vi "EOL CAN_Download CAL.vi"(4 "Download CAL Progress":refnum<vi>, 5 "Download CAL Time":refnum<vi>, 6 "ODX File Path":path, 7 "Tester":refnum<k21>, 8 "Error String":string, 9 "Glass?":bool=TRUE, 10 "Read Session in":refnum<k21>, 11 "DSC Write Session in":refnum<k21>) -> (1 "Error String Out":string, 2 "TxRx Data":string[][](array[string]), 3 "Response Good?":bool)   [LabVIEW 2014]
panel:
  in  "stop 2":bool
  in  "stop":bool
  out "error out":errorcluster
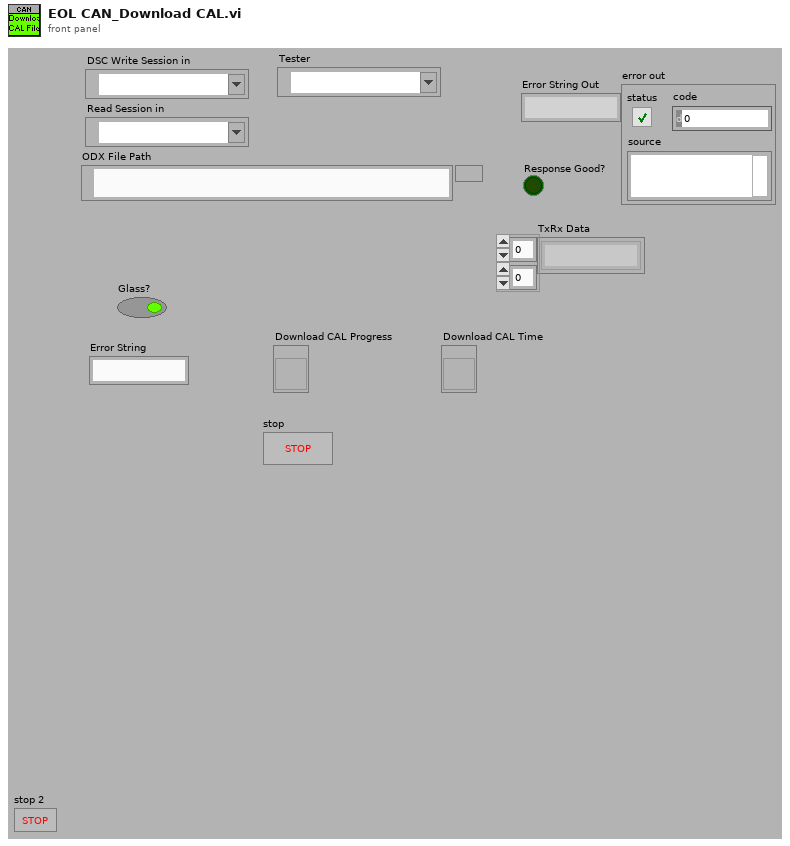
[diagram p1: front panel]
types:
  T1 = cluster{"DSC Write Session in":refnum<k21>, "Read Session in":refnum<k21>, "Error String":string, "Response Good?":bool, "Glass?":bool, "TxRx Data":string[][], "ODX File Path":path, "Flash Data Array":u8[], "Download CAL Progress":refnum<vi>, "Download CAL Time":refnum<vi>, "millisecond timer value":u32}
  T2 = typedef "Diagnose_SA2_Rechnenbefehl.ctl" = cluster{"Operation":T3, "Wert":u32}
  T3 = typedef "Diagnose_SA2_Operation_ENUM.ctl" = enum16{"RSL", "RSR", "ADD", "SUB", "EOR", "Durchläufe", "NEXT", "BCC", "BRA", "Fertig"}
  T4 = typedef "XNET Frame CAN.ctl" = cluster{"timestamp":timestamp, "payload":u8[], "identifier":u32, "type":T5, "extended?":bool, "echo?":bool}
  T5 = typedef "XNET Frame Type CAN.ctl" = u8
  T6 = cluster{"Start Adress":u8[], "Block Size":u8[], "Checksum":u8[]}
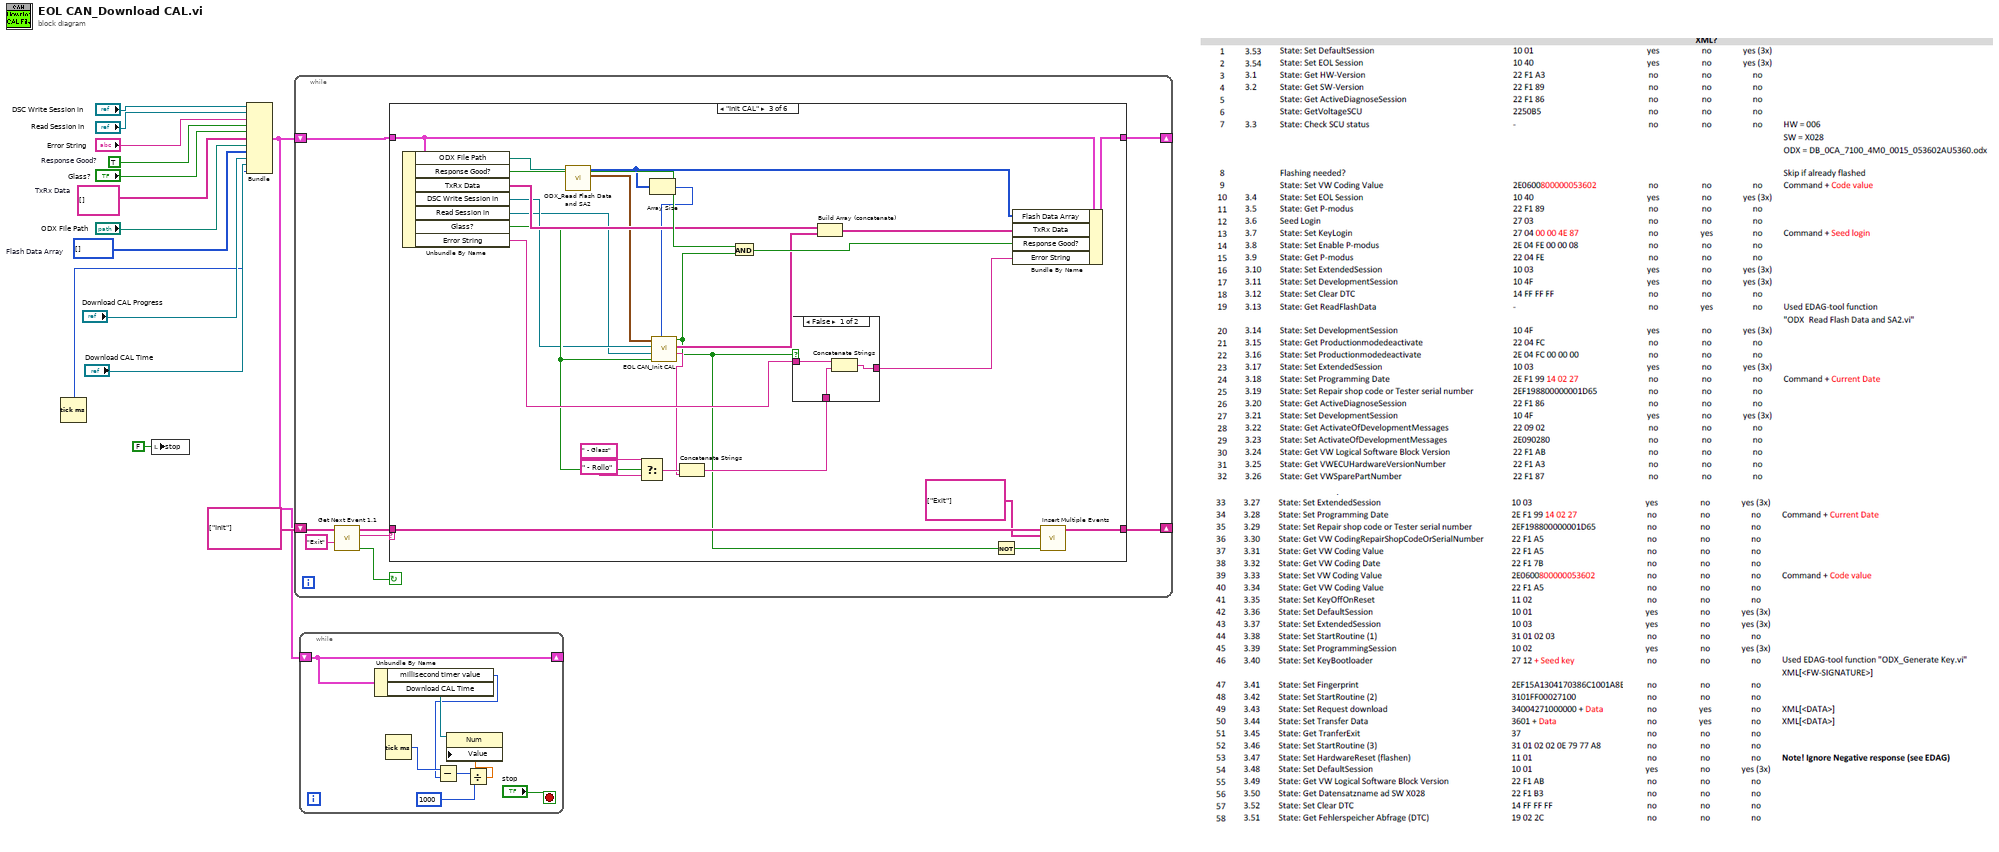
[diagram p0: block diagram]
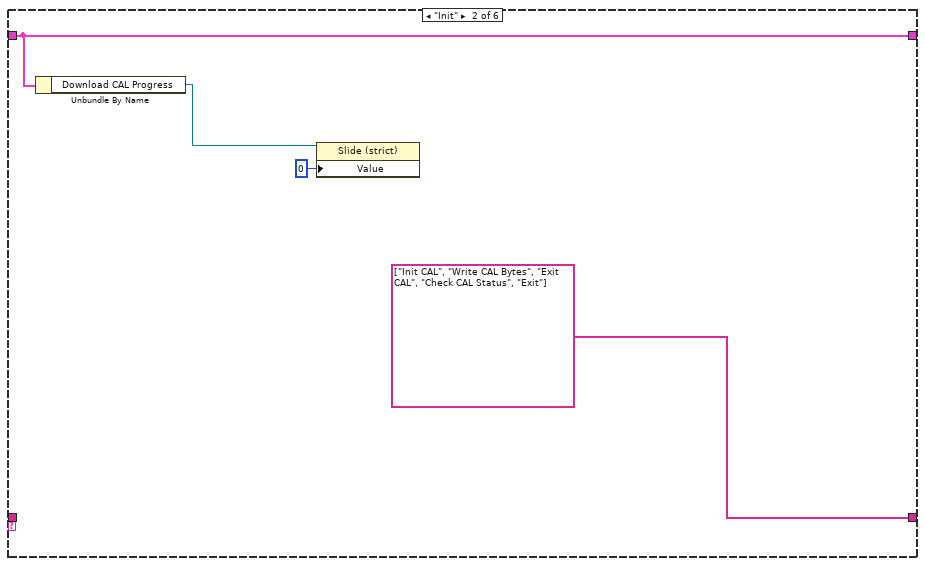
[diagram p3: hidden frame]
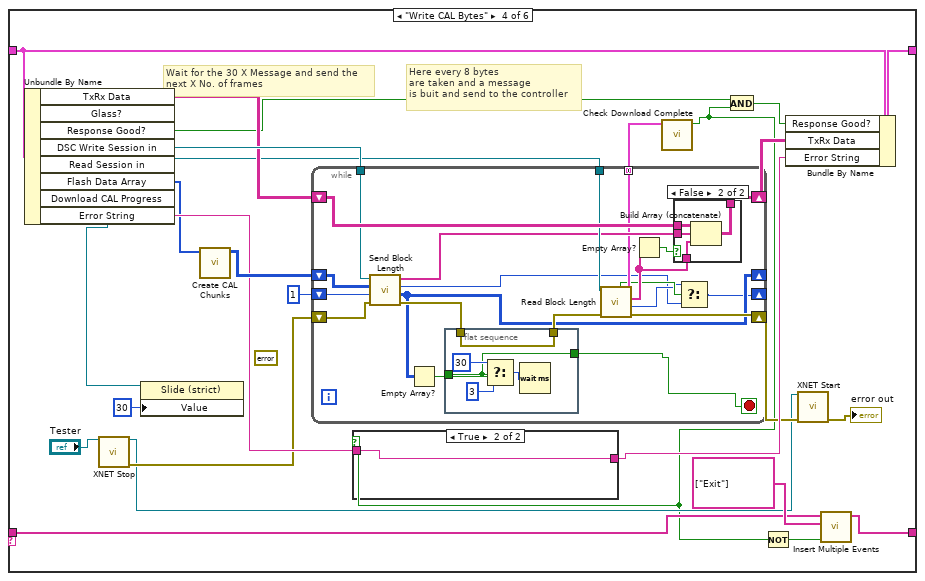
[diagram p5: hidden frame]
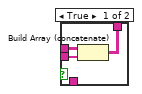
[diagram p6: hidden frame]
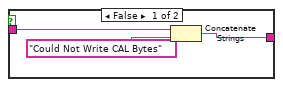
[diagram p7: hidden frame]
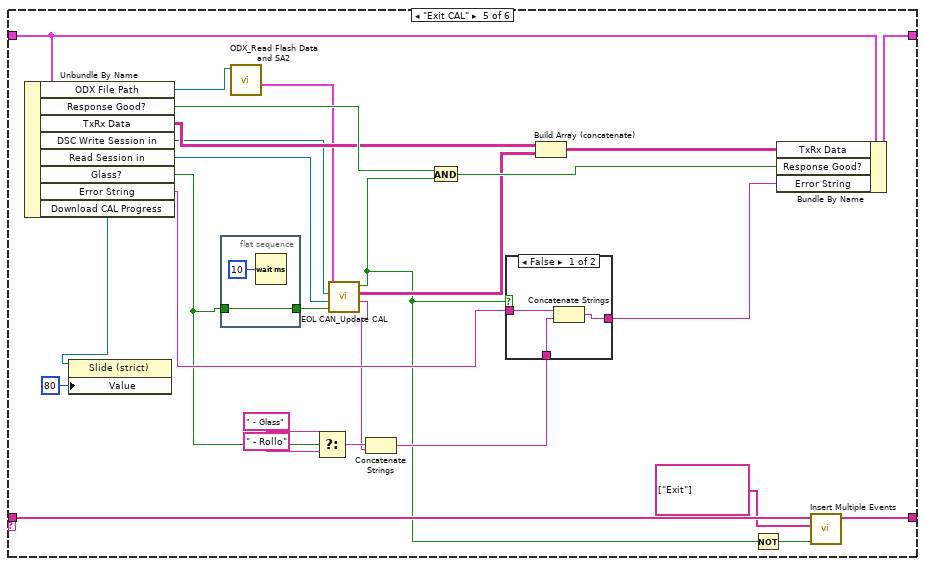
[diagram p8: hidden frame]
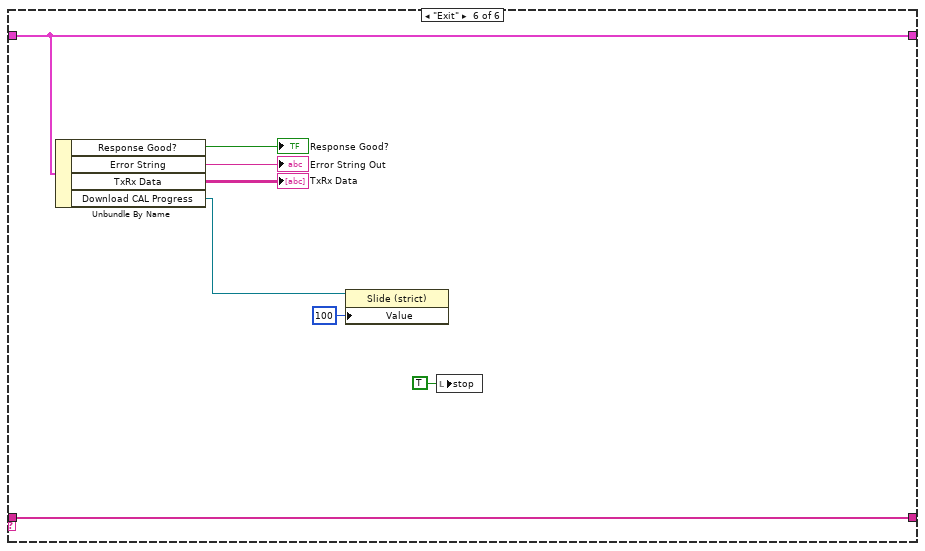
[diagram p10: hidden frame]
diagram:
  w6 = u8[] []  # Flash Data Array
  w10 = string[][] []  # TxRx Data
  w12 = TRUE  # Response Good?
  n1 = Tick Count (ms)() -> (millisecond timer value=w3:u32)
  n2 = local write "stop"(FALSE ("stop")) -> ()
  n3 = Bundle("DSC Write Session in"="DSC Write Session in", "Read Session in"="Read Session in", "Error String"="Error String", "Response Good?"=w12, "Glass?"="Glass?", "TxRx Data"=w10, "ODX File Path"="ODX File Path", "Flash Data Array"=w6, "Download CAL Progress"="Download CAL Progress", "Download CAL Time"="Download CAL Time", "millisecond timer value"=w3) -> (w2:T1)  [unwired: 1 in]
  n4 = while {
    shift-right: [w20] -> _
    shift-left: string[] ["Init"] ("event queue out") -> [w19]
    shift-right: [w18] -> _
    shift-left: w2 -> [w15]
    stop <- w22 continue-if-true
    n5 = call "Get Next Event 1.1.vi"("Exit Event"="Exit", "event queue in"=w19) -> ("Condition (Exit:F)"=w22:bool, "next event"=w16:string, "event queue out"=w21:string[])  [unwired: 6 in, 1 out]
    n6 = case shown="\"Init CAL\"" w16 {
      tunnel: w21 -> [w24 _ w43 w72 w145 w162]
      tunnel: [w24 string[] ["Init CAL", "Write CAL Bytes", "Exit CAL", "Check CAL Status", "Exit"] ("event queue out") w44 w73 w146 w162] -> w20
      tunnel: w15 -> [w23 w25 w53 w84 w148 w161]
      tunnel: [w23 w25 w51 w83 w147 w161] -> w18
      frame "Error", Default {
      }
      frame "Init" {
        n7 = Unbundle By Name(w25) -> ("Download CAL Progress"=w27:refnum<vi>)
        n8 = property class="Slide (strict)"(reference=w27, "Value"=u8 0) -> ()  [unwired: 1 in, 2 out]
      }
      frame "Init CAL" {
        n9 = Unbundle By Name(w53) -> ("ODX File Path"=w38:path, "Response Good?"=w54:bool, "TxRx Data"=w41:string[][], "DSC Write Session in"=w32:refnum<k21>, "Read Session in"=w31:refnum<k21>, "Glass?"=w33:bool, "Error String"=w50:string)
        n10 = call "ODX_Read Flash Data and SA2.vi"("ODX File Path"=w38) -> ("SA2 Operator"=w39:T2[], "Flash Data Array"=w30:u8[])  [unwired: 7 in, 2 out]
        n11 = Select(t=" - Glass" ("Error Description"), s=w33, f=" - Rollo" ("Error Description")) -> (s? t:f=w48:string)
        n12 = Array Size(array=w30) -> (size(s)=w29:i32)
        n13 = call "EOL CAN_Init CAL.vi"("Flash Size"=w29, "Glass?"=w33, "Read Session in"=w31, "DSC Write Session in"=w32, "SA2 Operator"=w39) -> ("Error String Out"=w36:string, "TxRx Data"=w37:string[][], "Response Good?"=w35:bool)  [unwired: 4 in]
        n14 = Concatenate Strings(w48, w36) -> (w45:string)
        n15 = And(x=w54, y=w35) -> (x .and. y?=w52:bool)
        n16 = case shown="False" w35 {
          tunnel: w50 -> [w56 w58]
          tunnel: [w57 w58] -> w49
          tunnel: w45 -> [w55 _]
          frame False {
            n17 = Concatenate Strings(w56, w55) -> (w57:string)
          }
          frame True {
          }
        }
        n18 = Build Array (concatenate)(w41, w37) -> (w40:string[][])
        n19 = Not(x=w35) -> (.not. x?=w34:bool)
        n20 = Bundle By Name(cluster=w53, "Flash Data Array"=w30, "TxRx Data"=w40, "Response Good?"=w52, "Error String"=w49) -> (w51:T1)
        n21 = call "Insert Multiple Events.vi"("Insert all? (T)"=w34, "Events to Insert"=string[] ["Exit"], "Event queue in"=w43) -> ("Event queue out"=w44:string[])  [unwired: 4 in]
      }
      frame "Write CAL Bytes" {
        (unwired) errorcluster {"status"=FALSE, "code"=0, "source"=""} ("error out 2")
        # "Wait for the 30 X Message and send the\nnext X No. of frames"
        # "Here every 8 bytes\nare taken and a message\nis buit and send to the controller"
        n22 = Unbundle By Name(w84) -> ("TxRx Data"=w81:string[][], "Response Good?"=w77:bool, "DSC Write Session in"=w82:refnum<k21>, "Read Session in"=w76:refnum<k21>, "Flash Data Array"=w59:u8[], "Download CAL Progress"=w70:refnum<vi>, "Error String"=w69:string)  [unwired: 1 out]
        n23 = call <vilib>:"XNET Stop.vi"("session in"="Tester") -> ("session out"=w64:refnum<k21>, "error out"=w66:errorcluster)  [unwired: 13 in]
        n24 = property class="Slide (strict)"(reference=w70, "Value"=u8 30) -> ()  [unwired: 1 in, 2 out]
        n25 = call "Create CAL Chunks.vi"("Flash Data Array"=w59) -> ("Array 2"=w80:u8[][])  [unwired: 10 in]
        n26 = while {
          tunnel: w82 -> [w103]
          shift-right: [w104] -> w79
          shift-left: w81 -> [w105]
          tunnel: w76 -> [w102]
          tunnel: [w100] -> w62 mode=concatenating
          shift-right: [w95] -> w65
          shift-left: w66 -> [w94]
          shift-right: [w86] -> _
          shift-left: u16 1 ("Block Size") -> [w93]
          shift-right: [w89] -> _
          shift-left: w80 -> [w91]
          stop <- w90 stop-if-true
          n27 = call "Send Block Length.vi"("error in (no error)"=w94, "Block Size In"=w93, "Array in"=w91, "Refnum in"=w103) -> ("error out"=w97:errorcluster, "Array Out"=w89:u8[][], "Block Size Out"=w85:u32, "Array out"=w101:string[])  [unwired: 4 in]
          n28 = Empty Array?(array=w89) -> (empty?=w92:bool)
          n29 = flat-sequence {
            tunnel: w97 -> [w110]
            tunnel: [w110] -> w96
            tunnel: w92 -> [w106]
            tunnel: [w106] -> w90
            frame #0 {
              n30 = Select(t=u32 30, s=w106, f=u32 3 ("milliseconds to wait")) -> (s? t:f=w109:u32)
              n31 = Wait (ms)(milliseconds to wait=w109) -> ()  [unwired: 1 out]
            }
          }
          n32 = call "Read Block Length.vi"("error in (no error)"=w96, "Refnum in"=w102) -> ("error out"=w95:errorcluster, "Block Size"=w87:u16, "Array"=w98:string[], "data"=w100:T4[], "Flow Control?"=w88:bool)  [unwired: 5 in]
          n33 = Empty Array?(array=w98) -> (empty?=w99:bool)
          n34 = case shown="False" w99 {
            tunnel: w105 -> [w113 w117]
            tunnel: [w112 w116] -> w104
            tunnel: w101 -> [w111 w115]
            tunnel: w98 -> [_ w114]
            frame True {
              n35 = Build Array (concatenate)(w113, w111) -> (w112:string[][])
            }
            frame False {
              n36 = Build Array (concatenate)(w117, w115, w114) -> (w116:string[][])
            }
          }
          n37 = Select(t=w87, s=w88, f=w85) -> (s? t:f=w86:u32)
        }
        n38 = call "Check Download Complete.vi"("data"=w62) -> ("Boolean"=w61:bool)  [unwired: 10 in]
        n39 = case shown="True" w61 {
          tunnel: w69 -> [w120 w121]
          tunnel: [w118 w121] -> w68
          frame False {
            n40 = Concatenate Strings(w120, "Could Not Write CAL Bytes" ("string")) -> (w118:string)
          }
          frame True {
          }
        }
        n41 = And(x=w77, y=w61) -> (x .and. y?=w78:bool)
        n42 = Not(x=w61) -> (.not. x?=w74:bool)
        n43 = Bundle By Name(cluster=w84, "Response Good?"=w78, "TxRx Data"=w79, "Error String"=w68) -> (w83:T1)
        n44 = call <vilib>:"XNET Start.vi"("session in"=w64, "error in (no error)"=w65) -> ("error out"=→"error out":errorcluster)  [unwired: 12 in, 1 out]
        n45 = call "Insert Multiple Events.vi"("Insert all? (T)"=w74, "Events to Insert"=string[] ["Exit"], "Event queue in"=w72) -> ("Event queue out"=w73:string[])  [unwired: 4 in]
      }
      frame "Exit CAL" {
        n46 = Unbundle By Name(w148) -> ("ODX File Path"=w127:path, "Response Good?"=w144:bool, "TxRx Data"=w135:string[][], "DSC Write Session in"=w132:refnum<k21>, "Read Session in"=w131:refnum<k21>, "Glass?"=w125:bool, "Error String"=w142:string, "Download CAL Progress"=w122:refnum<vi>)
        n47 = property class="Slide (strict)"(reference=w122, "Value"=u8 80) -> ()  [unwired: 1 in, 2 out]
        n48 = flat-sequence {
          tunnel: w125 -> [w149]
          tunnel: [w149] -> w124
          frame #0 {
            n49 = Wait (ms)(milliseconds to wait=u32 10) -> ()  [unwired: 1 out]
          }
        }
        n50 = call "ODX_Read Flash Data and SA2.vi"("ODX File Path"=w127) -> ("Download Parameter"=w126:T6)  [unwired: 7 in, 3 out]
        n51 = Select(t=" - Glass" ("Error Description"), s=w125, f=" - Rollo" ("Error Description")) -> (s? t:f=w140:string)
        n52 = call "EOL CAN_Update CAL.vi"("Glass?"=w124, "Read Session in"=w131, "DSC Write Session in"=w132, "Download Parameter"=w126) -> ("Error String Out"=w129:string, "TxRx Data"=w130:string[][], "Response Good?"=w128:bool)  [unwired: 5 in]
        n53 = Concatenate Strings(w140, w129) -> (w137:string)
        n54 = And(x=w144, y=w128) -> (x .and. y?=w143:bool)
        n55 = case shown="False" w128 {
          tunnel: w142 -> [w152 w154]
          tunnel: [w153 w154] -> w141
          tunnel: w137 -> [w151 _]
          frame False {
            n56 = Concatenate Strings(w152, w151) -> (w153:string)
          }
          frame True {
          }
        }
        n57 = Build Array (concatenate)(w135, w130) -> (w134:string[][])
        n58 = Not(x=w128) -> (.not. x?=w133:bool)
        n59 = Bundle By Name(cluster=w148, "TxRx Data"=w134, "Response Good?"=w143, "Error String"=w141) -> (w147:T1)
        n60 = call "Insert Multiple Events.vi"("Insert all? (T)"=w133, "Events to Insert"=string[] ["Exit"], "Event queue in"=w145) -> ("Event queue out"=w146:string[])  [unwired: 4 in]
      }
      frame "Exit" {
        n61 = Unbundle By Name(w161) -> ("Response Good?"=→"Response Good?":bool, "Error String"=→"Error String Out":string, "TxRx Data"=→"TxRx Data":string[][], "Download CAL Progress"=w156:refnum<vi>)
        n62 = property class="Slide (strict)"(reference=w156, "Value"=u8 100) -> ()  [unwired: 1 in, 2 out]
        n63 = local write "stop"(TRUE ("stop")) -> ()
      }
    }
  }
  n64 = while {
    shift-right: [w165] -> _
    shift-left: w2 -> [w165]
    stop <- "stop" stop-if-true
    n65 = Unbundle By Name(w165) -> ("millisecond timer value"=w164:u32, "Download CAL Time"=w169:refnum<vi>)
    n66 = Tick Count (ms)() -> (millisecond timer value=w166:u32)
    n67 = Subtract(x=w166, y=w164) -> (x-y=w167:u32)
    n68 = Divide(x=w167, y=u32 1000) -> (x/y=w170:dbl)
    n69 = property class="Num"(reference=w169, "Value"=w170) -> ()  [unwired: 1 in, 2 out]
  }
